vi "Clear Components.vi"(8 "error in (no error)":errorcluster, 11 "Blueprint in":refnum<class "Blueprint.lvclass">) -> (0 "error out":errorcluster, 3 "Blueprint out":refnum<class "Blueprint.lvclass">)   [LabVIEW 2020, in "Blueprint.lvclass"]
uses:
  Blueprint.lvclass
  Blueprint.lvclass/Blueprint.ctl
  Item/Ingredient.ctl
  Item/Item.lvclass
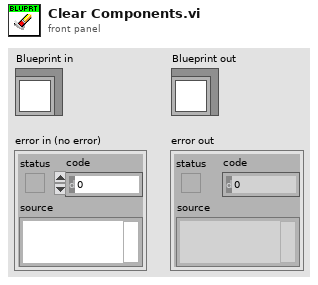
[diagram p1: front panel]
types:
  T1 = typedef "Item.lvclass/Ingredient.ctl" = cluster{"Item":refnum<class "Item.lvclass">, "Qty":dbl}
  T2 = typedef "Blueprint.lvclass/Ref Data.ctl" = cluster{"Ingredients":T1[], "Workstation":refnum<class "Workstation.lvclass">, "Craft Time":dbl, "Name":string}
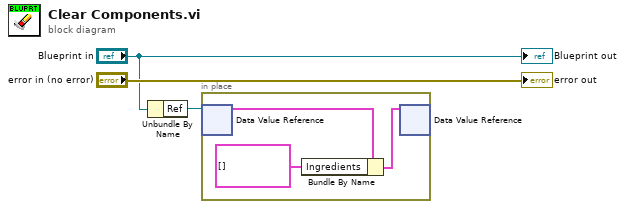
[diagram p0: block diagram]
diagram:
  n1 = Unbundle By Name("Blueprint in") -> ("Ref"=w2:refnum<data-value>)
  n2 = in-place {
    n3 = in-place-dvr #1(w2) -> (w6:T2)  [unwired: 1 out]
    n4 = Bundle By Name(cluster=w6, "Ingredients"=T1[] []) -> (w5:T2)
    n5 = in-place-dvr #1(w5) -> ()  [unwired: 2 out]
  }
  "error out" <- "error in (no error)"
  "Blueprint out" <- "Blueprint in"
